vi "Configure Power Setpoint.vi"(8 "error in (no error)":errorcluster, 9 "Power Setpoint (0 watts)":dbl, 10 "Power Setpoint Type (0: Minimum)":i32(ring) items=["Minimum", "Maximum", "Value"], 11 "VISA resource name":refnum<visa-resource-name>) -> (0 "error out":errorcluster, 3 "VISA resource name out":refnum<visa-resource-name>)   [LabVIEW 2018, in "XP Power PLS600.lvlib"]
doc: "Configures the output power setpoint as specified. The setpoint can be set to minimum, maximum, or a specified value in watts. \n<b>NOTE</b>: The System Mode must be set to Remote before using this function."
uses:
  XP Power PLS600.lvlib
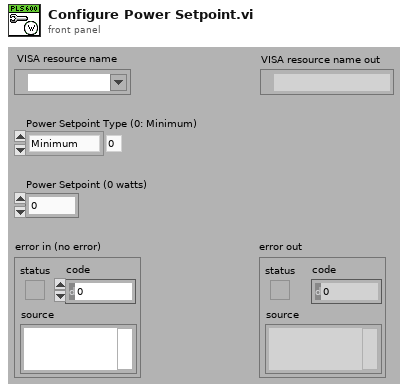
[diagram p1: front panel]
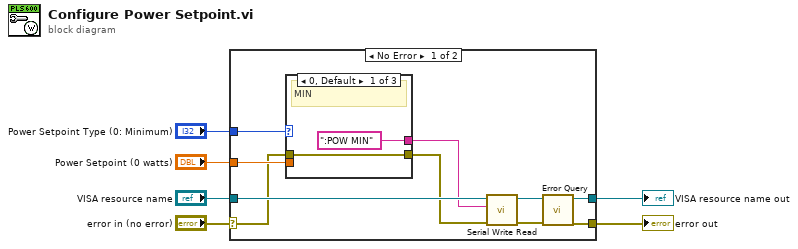
[diagram p0: block diagram]
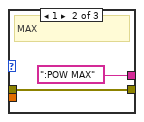
[diagram p2: hidden frame]
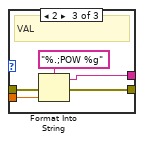
[diagram p3: hidden frame]
diagram:
  n1 = case shown="No Error" "error in (no error)" {
    selector: "error in (no error)" -> [w7 w26]
    tunnel: [w16 w27] -> w6
    tunnel: [w15 w26] -> w5
    tunnel: "Power Setpoint (0 watts)" -> [w14 _]
    tunnel: "Power Setpoint Type (0: Minimum)" -> [w13 _]
    tunnel: "VISA resource name" -> [w12 w27]
    frame No Error {
      n2 = case shown="0, Default" w13 {
        tunnel: [":POW MIN" ":POW MAX" w24] -> w10
        tunnel: w14 -> [_ _ w23]
        tunnel: w7 -> [w17 w19 w22]
        tunnel: [w17 w19 w21] -> w11
        frame 0, Default {
          # "MIN"
        }
        frame 1 {
          # "MAX"
        }
        frame 2 {
          # "VAL"
          n3 = Format Into String(format string="%.;POW %g", error in=w22, w23) -> (resulting string=w24:string, error out=w21:errorcluster)  [unwired: 1 in]
        }
      }
      n4 = call "Serial Write Read.vi"("error in (no error)"=w11, "Write Buffer"=w10, "VISA resource name"=w12) -> ("error out"=w8:errorcluster, "VISA resource name out"=w9:refnum<visa-resource-name>)  [unwired: 6 in, 1 out]
      n5 = call "Error Query.vi"("error in (no error)"=w8, "VISA resource name"=w9) -> ("error out"=w15:errorcluster, "VISA resource name out"=w16:refnum<visa-resource-name>)  [unwired: 6 in, 2 out]
    }
    frame Error {
    }
  }
  "VISA resource name out" <- w6
  "error out" <- w5
